vi "Acquisition Started.vi"(8 "error in (no error)":errorcluster, 10 "Reply Payload":T1) -> (0 "error out":errorcluster)   [LabVIEW 2018, in "LGP5 Acquisition.lvlib"]
doc: "The Start Acquiring request event requests the module to configure the DAQ device and start acquiring.\nThe Acquisition Started broadcast event indicates when the DAQ device has started aquiring.\n_____\nCreated using Delacor QMH Event Scripter 4.2.0.84."
uses:
  LGP5 Acquisition.lvlib
  Start Acquiring (Reply Payload)--cluster.ctl
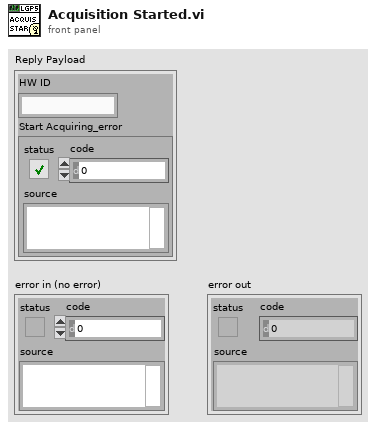
[diagram p1: front panel]
types:
  T1 = typedef "LGP5 Acquisition.lvlib/Start Acquiring (Reply Payload)--cluster.ctl" = cluster{"HW ID":string, "Start Acquiring_error":errorcluster}
  T2 = typedef "LGP5 Acquisition.lvlib/Broadcast Events--cluster.ctl" = cluster{"Module Did Init":refnum<user-event>, "Status Updated":refnum<user-event>, "Error Reported":refnum<user-event>, "Module Did Stop":refnum<user-event>, "Update Module Execution Status":refnum<user-event>, "Acquisition Started":refnum<user-event>}
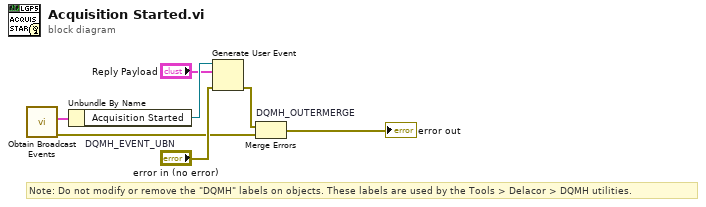
[diagram p0: block diagram]
diagram:
  # "Note: Do not modify or remove the \"DQMH\" labels on objects. These labels are used by the Tools > Delacor > DQMH utilities."
  n1 = call "Obtain Broadcast Events.vi"() -> ("error out"=w3:errorcluster, "LGP5 Acquisition Broadcast Events"=w2:T2)  [unwired: 10 in]
  n2 = Unbundle By Name "DQMH_EVENT_UBN"(w2) -> ("Acquisition Started"=w5:refnum<user-event>)
  n3 = Generate User Event(user event=w5, event data cluster="Reply Payload", error in="error in (no error)") -> (error out=w4:errorcluster)  [unwired: 1 in, 1 out]
  n4 = Merge Errors "DQMH_OUTERMERGE"(w4, w3) -> (→"error out":errorcluster)
